vi "Generic Camera Wait For New Frame Ref.vi"(0 "Image Ref":T1, 11 "Error In":errorcluster, 13 "Wait No. (1)":u32=1) -> (4 "Image Ref Out":T1, 15 "Error Out":errorcluster)   [LabVIEW 2025]
uses:
  <vilib>/vision/Image Controls.llb/IMAQ Image.ctl
  Camera Controls/Camera IMAQ Key Info.ctl
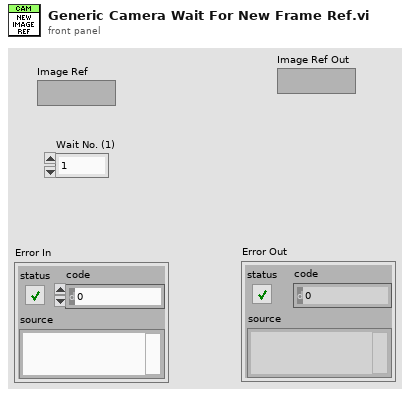
[diagram p1: front panel]
types:
  T1 = typedef "IMAQ Image.ctl" = refnum<image>
  T2 = typedef "Camera IMAQ Key Info.ctl" = cluster{"Frame":u32, "Sensor Height":i32, "Sensor Width":i32, "ROI Height":i32, "ROI Width":i32, "ROI Enable?":bool, "Bit per Pixel":u8}
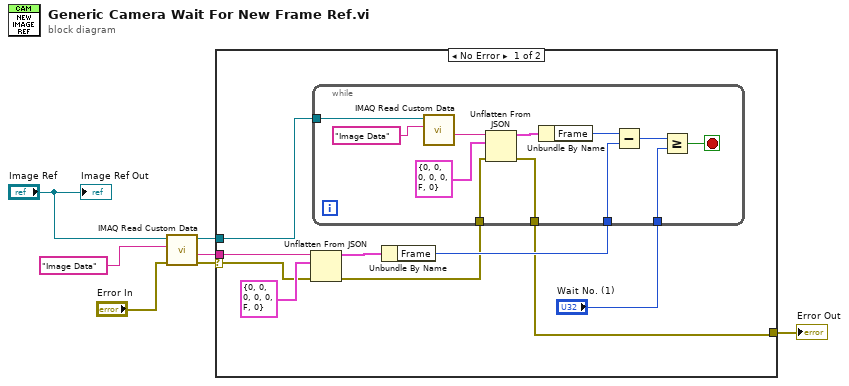
[diagram p0: block diagram]
diagram:
  n1 = call "IMAQ Read Custom Data"("error in (no error)"="Error In", "Key"="Image Data", "Image"="Image Ref") -> ("error out"=w4:errorcluster, "Custom Data Out"=w7:string, "Image (duplicate)"=w5:T1)  [unwired: 6 in]
  n2 = case shown="No Error" w4 {
    selector: w4 -> [w10 w29]
    tunnel: w7 -> [w14 _]
    tunnel: w5 -> [w13 _]
    tunnel: [w8 w29] -> w1
    frame No Error {
      n3 = Unflatten From JSON(JSON string=w14, type and defaults=T2 {"Frame"=0, "Sensor Height"=0, "Sensor Width"=0, "ROI Height"=0, "ROI Width"=0, "ROI Enable?"=FALSE, "Bit per Pixel"=0} ("Camera IMAQ Key Info"), error in (no error)=w10) -> (value=w16:T2, error out=w9:errorcluster)  [unwired: 4 in]
      n4 = Unbundle By Name(w16) -> ("Frame"=w12:u32)
      n5 = while {
        tunnel: w13 -> [w24]
        tunnel: w12 -> [w22]
        tunnel: "Wait No. (1)" -> [w19]
        tunnel: w9 -> [w18]
        tunnel: [w17] -> w8
        stop <- w20 stop-if-true
        n6 = call "IMAQ Read Custom Data"("Key"="Image Data", "Image"=w24) -> ("Custom Data Out"=w26:string)  [unwired: 7 in, 2 out]
        n7 = Unflatten From JSON(JSON string=w26, type and defaults=T2 {"Frame"=0, "Sensor Height"=0, "Sensor Width"=0, "ROI Height"=0, "ROI Width"=0, "ROI Enable?"=FALSE, "Bit per Pixel"=0} ("Camera IMAQ Key Info"), error in (no error)=w18) -> (value=w28:T2, error out=w17:errorcluster)  [unwired: 4 in]
        n8 = Unbundle By Name(w28) -> ("Frame"=w23:u32)
        n9 = Subtract(x=w23, y=w22) -> (x-y=w21:u32)
        n10 = Greater Or Equal?(x=w21, y=w19) -> (x >= y?=w20:bool)
      }
    }
    frame Error {
    }
  }
  "Error Out" <- w1
  "Image Ref Out" <- "Image Ref"
